vi "uActor_Core.vi"(8 "error in (no error)":errorcluster, 11 "uActor in":refnum<class "uActor.lvclass">) -> (0 "error out":errorcluster, 3 "uActor out":refnum<class "uActor.lvclass">)   [LabVIEW 2023, in "uLib.lvlib" / "uActor.lvclass"]
doc: "Dynamic dispatch method to allow children to add helper loops when desired."
uses:
  uActor.lvclass
  uActor.lvclass/uActor.ctl
  uTransport/uTransport_uActor/uTransport_uActor.lvclass/uTransport_uActor.ctl
  uMsg/uMsg/uMsg.lvclass/uMsg.ctl
  uMsg/uMsg/uMsg.lvclass
  uData/uData/uData.lvclass/uData.ctl
  uData/uData/Condition Tag Name.vi
  uActor_Get Self Transport.vi
  uData/uData/Combine Tags.vi
  uTransport/uTransport/uTransport_SendMsg.vi
  uData/uData/Blank Key Reserved String.vi
  uMsg/uMsg/uMsg Update Timestamp.vi
  uData/uData/uData.lvclass
  uTransport/uTransport/uTransport.lvclass
  uErr/uErr/uErr.lvclass
  uTransport/uTransport_uActor/uTransport_uActor.lvclass
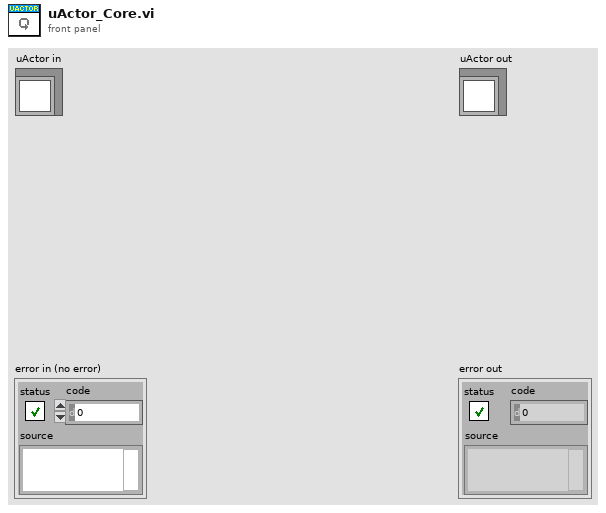
[diagram p1: front panel]
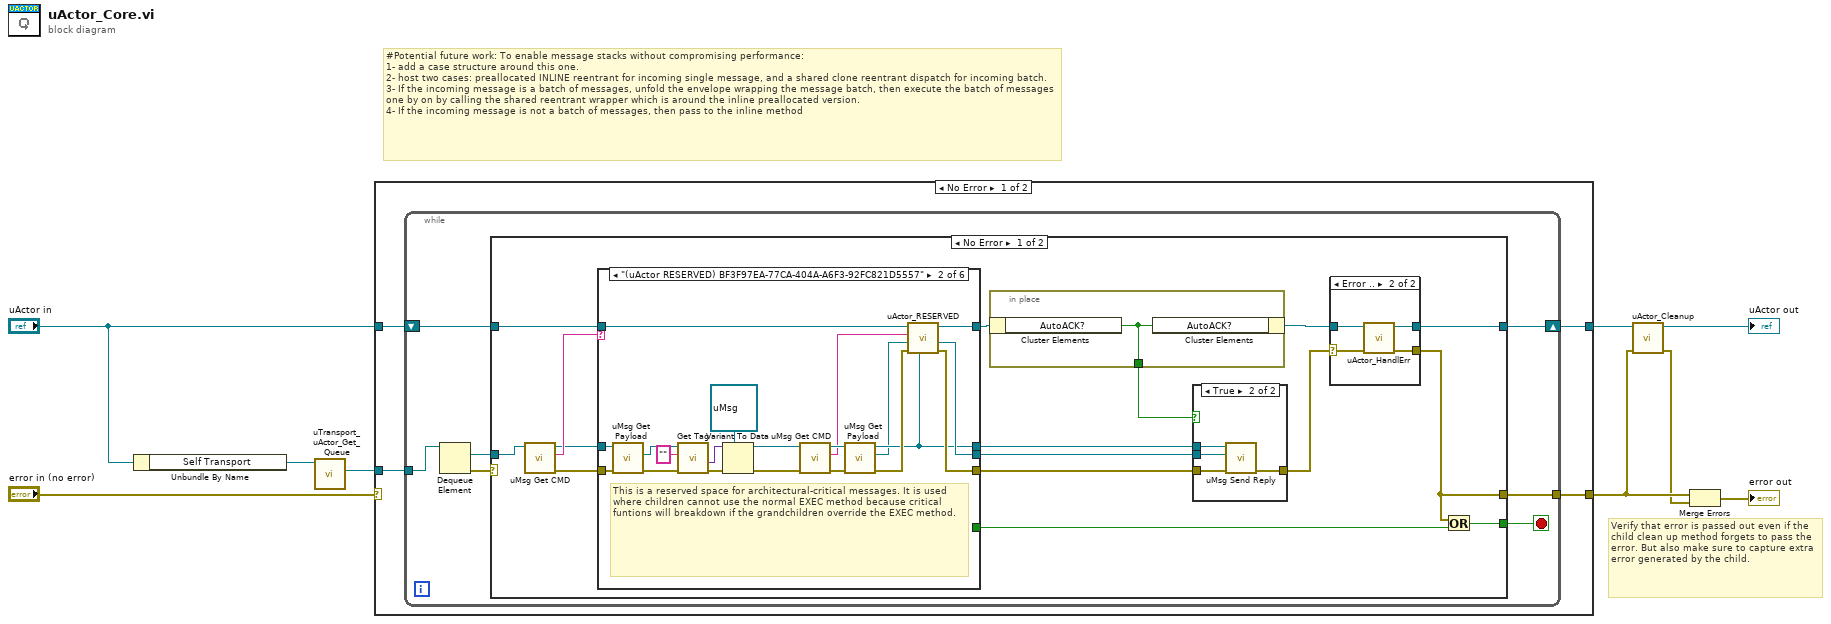
[diagram p0: block diagram]
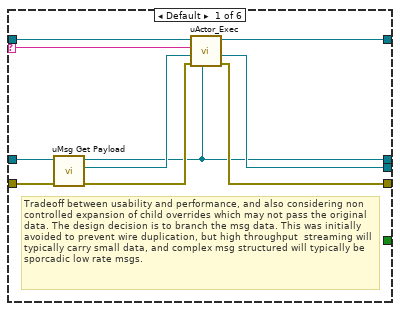
[diagram p2: hidden frame]
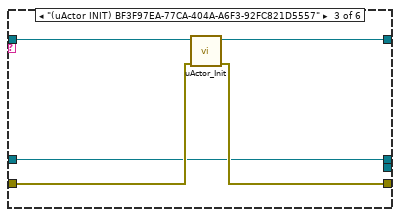
[diagram p3: hidden frame]
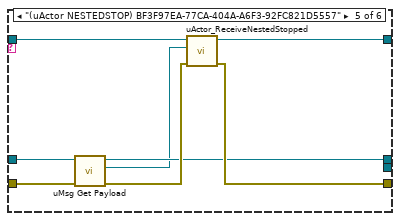
[diagram p5: hidden frame]
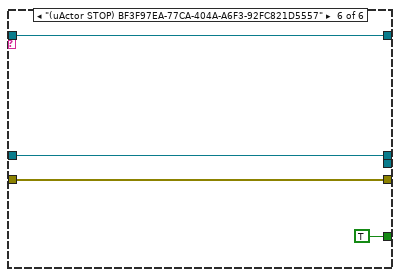
[diagram p6: hidden frame]
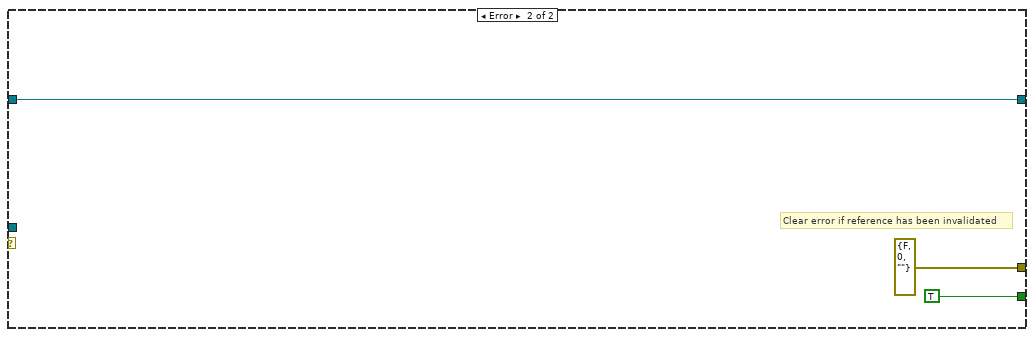
[diagram p9: hidden frame]
diagram:
  # "Verify that error is passed out even if the child clean up method forgets to pass the error. But also make sure to capture extra error generated by the child."
  # "#Potential future work: To enable message stacks without compromising performance:\n1- add a case structure around this one. \n2- host two cases: preallocated INLINE reentrant for incoming single message, and a shared clone reentrant dispatch for incoming batch.\n3- If the incoming message is a batch of messages, unfold the envelope wrapping the message batch, then execute the batch of messages one by on by calling the shared reentrant wrapper which is around the inline preallocated version.\n4- If the incoming message is not a batch of messages, then pass to the inline method"
  n1 = Unbundle By Name("uActor in") -> ("Self Transport"=w8:refnum<class "uTransport_uActor.lvclass">)
  n2 = call "uTransport_uActor_Get_Queue.vi"("uTransport_uActor in"=w8) -> ("Actor Queue"=w7:refnum<queue>)  [unwired: 10 in]
  n3 = case shown="No Error" "error in (no error)" {
    selector: "error in (no error)" -> [_ w103]
    tunnel: [w10 w103] -> w3
    tunnel: [w13 w102] -> w6
    tunnel: "uActor in" -> [w12 w102]
    tunnel: w7 -> [w11 _]
    frame No Error {
      n4 = while {
        shift-right: [w17] -> w13
        shift-left: w12 -> [w19]
        tunnel: w11 -> [w20]
        tunnel: [w15] -> w10
        stop <- w16 stop-if-true
        n5 = Dequeue Element(queue=w20) -> (element=w18:refnum<class "uMsg.lvclass">, error out=w14:errorcluster)  [unwired: 2 in, 2 out]
        n6 = case shown="No Error" w14 {
          tunnel: w19 -> [w35 w99]
          tunnel: w18 -> [w34 _]
          tunnel: [w32 w99] -> w17
          tunnel: [w31 TRUE] -> w16
          tunnel: [w30 errorcluster {"status"=FALSE, "code"=0, "source"=""} ("error out")] -> w15
          frame No Error {
            n7 = call "uMsg Get CMD.vi"("uMsg in"=w34) -> ("error out"=w36:errorcluster, "CMD"=w33:string, "uMsg out"=w26:refnum<class "uMsg.lvclass">)  [unwired: 8 in]
            n8 = case shown="\"(uActor RESERVED) BF3F97EA-77CA-404A-A6F3-92FC821D5557\"" w33 {
              selector: w33 -> [w44 _ _ _ _ _]
              tunnel: [w45 w65 w70 w74 w81 w85] -> w28
              tunnel: w36 -> [w41 w63 w69 w74 w78 w85]
              tunnel: [w47 w67 w72 w75 w82 w86] -> w23
              tunnel: w35 -> [w46 w66 w71 w75 w83 w86]
              tunnel: w26 -> [w40 w62 w68 w73 w80 w84]
              tunnel: [_ _ _ _ _ TRUE] -> w29
              tunnel: [w43 w64 _ _ _ _] -> w27
              tunnel: [w38 w53 w68 w73 w77 w84] -> w25
              frame Default {
                # "Tradeoff between usability and performance, and also considering non controlled expansion of child overrides which may not pass the original data. The design decision is to branch the msg data. This was initially avoided to prevent wire duplication, but high throughput  streaming will typically carry small data, and complex msg structured will typically be sporcadic low rate msgs."
                n9 = call "uMsg Get Payload.vi"("error in (no error)"=w41, "uMsg in"=w40) -> ("error out"=w42:errorcluster, "uData"=w39:refnum<class "uData.lvclass">, "uMsg out"=w38:refnum<class "uMsg.lvclass">)  [unwired: 7 in]
                n10 = call-dynamic "uActor_Exec.vi"("Original uMsg"=w38, "error in (no error)"=w42, "Data"=w39, "Command"=w44, "uActor in"=w46) -> ("error out"=w45:errorcluster, "reply"=w43:refnum<class "uData.lvclass">, "uActor out"=w47:refnum<class "uActor.lvclass">)  [unwired: 4 in]
              }
              frame "(uActor RESERVED) BF3F97EA-77CA-404A-A6F3-92FC821D5557" {
                # "This is a reserved space for architectural-critical messages. It is used where children cannot use the normal EXEC method because critical funtions will breakdown if the grandchildren override the EXEC method."
                n11 = call "uMsg Get Payload.vi"("error in (no error)"=w63, "uMsg in"=w62) -> ("error out"=w61:errorcluster, "uData"=w59:refnum<class "uData.lvclass">)  [unwired: 7 in, 1 out]
                n12 = call "Get Tag.vi"("error in (no error)"=w61, "tag (case insensitive)"="", "uData in"=w59) -> ("error out"=w60:errorcluster, "value"=w57:variant)  [unwired: 5 in, 2 out]
                n13 = Variant To Data(error in=w60, type=refnum<class "uMsg.lvclass"> refnum ("uMsg out"), Variant=w57) -> (data=w50:refnum<class "uMsg.lvclass">, error out=w55:errorcluster)
                n14 = call "uMsg Get CMD.vi"("error in (no error)"=w55, "uMsg in"=w50) -> ("error out"=w51:errorcluster, "CMD"=w48:string, "uMsg out"=w49:refnum<class "uMsg.lvclass">)  [unwired: 7 in]
                n15 = call "uMsg Get Payload.vi"("error in (no error)"=w51, "uMsg in"=w49) -> ("error out"=w54:errorcluster, "uData"=w52:refnum<class "uData.lvclass">, "uMsg out"=w53:refnum<class "uMsg.lvclass">)  [unwired: 7 in]
                n16 = call-dynamic "uActor_RESERVED.vi"("Original uMsg"=w53, "error in (no error)"=w54, "Data"=w52, "Command"=w48, "uActor in"=w66) -> ("error out"=w65:errorcluster, "reply"=w64:refnum<class "uData.lvclass">, "uActor out"=w67:refnum<class "uActor.lvclass">)  [unwired: 4 in]
              }
              frame "(uActor INIT) BF3F97EA-77CA-404A-A6F3-92FC821D5557" {
                n17 = call-dynamic "uActor_Init.vi"("error in (no error)"=w69, "uActor in"=w71) -> ("error out"=w70:errorcluster, "uActor out"=w72:refnum<class "uActor.lvclass">)  [unwired: 8 in]
              }
              frame "(uActor NULL) BF3F97EA-77CA-404A-A6F3-92FC821D5557" {
                # "Children may NOT override the blank string behavior. It invokes the the NULL case. Blank strings are part of the reserved non-overridable framework functions"
                # "Blank string received, or intentional NULL msg."
              }
              frame "(uActor NESTEDSTOP) BF3F97EA-77CA-404A-A6F3-92FC821D5557" {
                n18 = call "uMsg Get Payload.vi"("error in (no error)"=w78, "uMsg in"=w80) -> ("error out"=w79:errorcluster, "uData"=w76:refnum<class "uData.lvclass">, "uMsg out"=w77:refnum<class "uMsg.lvclass">)  [unwired: 7 in]
                n19 = call "uActor_ReceiveNestedStopped.vi"("error in (no error)"=w79, "uData in"=w76, "uActor in"=w83) -> ("error out"=w81:errorcluster, "uActor out"=w82:refnum<class "uActor.lvclass">)  [unwired: 7 in]
              }
              frame "(uActor STOP) BF3F97EA-77CA-404A-A6F3-92FC821D5557" {
              }
            }
            n20 = in-place {
              in-place-border: [w37] -> w21
              n21 = in-place-cluster #1(w23) -> ("AutoACK?"=w37:bool)
              n22 = in-place-cluster #1("AutoACK?"=w37) -> (w22:refnum<class "uActor.lvclass">)
            }
            n23 = case shown="True" w21 {
              tunnel: w28 -> [w88 w92]
              tunnel: w27 -> [_ w91]
              tunnel: w25 -> [_ w89]
              tunnel: [w88 w90] -> w24
              frame False {
              }
              frame True {
                n24 = call "uMsg Send Reply.vi"("error in (no error)"=w92, "Reply Data"=w91, "Original Msg"=w89) -> ("error out"=w90:errorcluster)  [unwired: 8 in]
              }
            }
            n25 = case shown="Error .." w24 {
              selector: w24 -> [w93 w96]
              tunnel: w22 -> [w94 w98]
              tunnel: [w94 w97] -> w32
              tunnel: [w93 w95] -> w30
              frame No Error {
              }
              frame Error {
                n26 = call "uActor_HandlErr.vi"("error in (no error)"=w96, "uActor in"=w98) -> ("error out"=w95:errorcluster, "uActor out"=w97:refnum<class "uActor.lvclass">)  [unwired: 8 in]
              }
            }
            n27 = Or(x=w30, y=w29) -> (x .or. y?=w31:bool)
          }
          frame Error {
            # "Clear error if reference has been invalidated"
          }
        }
      }
    }
    frame Error {
    }
  }
  n28 = call-dynamic "uActor_Cleanup.vi"("error in (no error)"=w3, "uActor in"=w6) -> ("error out"=w2:errorcluster, "uActor out"=→"uActor out":refnum<class "uActor.lvclass">)  [unwired: 8 in]
  n29 = Merge Errors(w3, w2) -> (→"error out":errorcluster)
